vi "Convert (tau, f) to (jw, z).vi"(9 "Harmonic Frequency":dbl[unit], 10 "Lifetime":dbl[unit]) -> (1 "Phasor":cdb, 2 "i 2 pi f (GHz)":cdb)   [LabVIEW 2019]
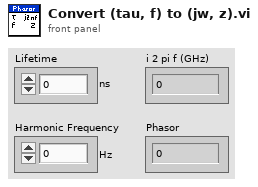
[diagram p1: front panel]
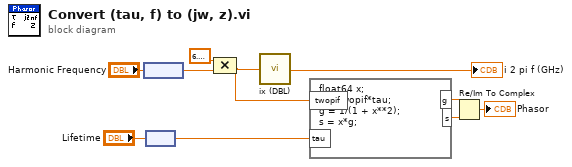
[diagram p0: block diagram]
diagram:
  n1 = node("Harmonic Frequency") -> (w4:dbl)
  n2 = node("Lifetime") -> (w3:dbl)
  n3 = Compound Arithmetic op=MULTIPLY(6.283185307179586, w4) -> (w2:dbl)
  n4 = call "ix (DBL).vi"("x (1)"=w2) -> ("i.(x)"=→"i 2 pi f (GHz)":cdb)
  n5 = formula code="float64 x;\nx = twopif*tau;\ng = 1/(1 + x**2);\ns = x*g;"("twopif"=w2, "tau"=w3) -> ("g"=w6:dbl, "s"=w7:dbl)
  n6 = Re/Im To Complex(1:w7, 2:w6) -> (0:→"Phasor":cdb)
